vi "Remote.vi"(0 "VISA resource name":refnum<visa-resource-name>, 5 "Remote (F: Local)":bool, 11 "error in (no error)":errorcluster) -> (4 "VISA resource name out":refnum<visa-resource-name>, 15 "error out":errorcluster)   [LabVIEW 2013, in "Yokogawa WT200 Series.lvlib"]
doc: "This VI sends the Remote command to the WT200 Series.\n\nNote : This VI is used for the Serial Interface."
uses:
  <instrlib>/Yokogawa WT200 Series/Yokogawa WT200 Series.lvlib
panel:
  # "Remote\nLocal"
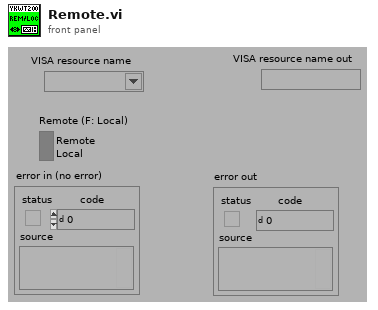
[diagram p1: front panel]
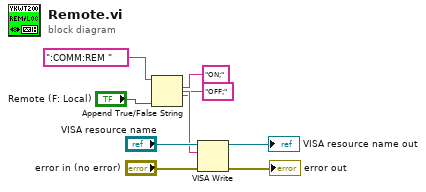
[diagram p0: block diagram]
diagram:
  n1 = Append True/False String(1:"Remote (F: Local)", 2:"OFF;", 3:"ON;", 4:":COMM:REM ") -> (0:w5:string)
  n2 = VISA Write(VISA resource name="VISA resource name", write buffer=w5, error in (no error)="error in (no error)") -> (VISA resource name out=→"VISA resource name out":refnum<visa-resource-name>, error out=→"error out":errorcluster)  [unwired: 1 out]
